vi "Stats to % Passing.vi"(11 "Stats by Ranking":T2) -> (3 "% Passing":T1)   [LabVIEW 2023, in "VIA Results Handling.lvlib"]
doc: "Converts stats by ranking into a % Passing by ranking."
uses:
  VIA Results Handling.lvlib
  Stats by Ranking.ctl
  Stats Cluster.ctl
  Ranking Percent Passing Cluster.ctl
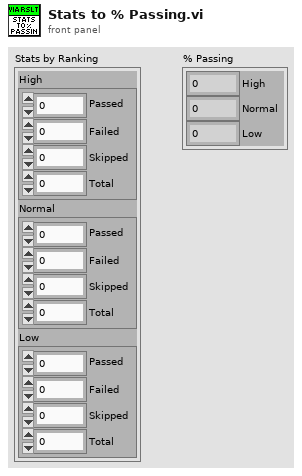
[diagram p1: front panel]
types:
  T1 = typedef "VIA Results Handling.lvlib/Ranking Percent Passing Cluster.ctl" = cluster{"High":dbl, "Normal":dbl, "Low":dbl}
  T2 = typedef "VIA Results Handling.lvlib/Stats by Ranking.ctl" = cluster{"High":T3, "Normal":T3, "Low":T3}
  T3 = typedef "VIA Results Handling.lvlib/Stats Cluster.ctl" = cluster{"Passed":i32, "Failed":i32, "Skipped":i32, "Total":i32}
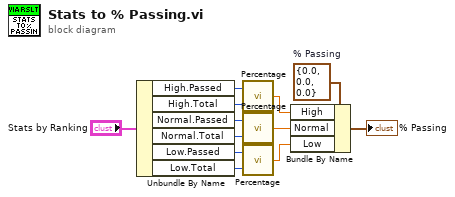
[diagram p0: block diagram]
diagram:
  w7 = T1 {"High"=0.0, "Normal"=0.0, "Low"=0.0}  # % Passing
  n1 = Unbundle By Name("Stats by Ranking") -> ("High.Passed"=w2:i32, "High.Total"=w1:i32, "Normal.Passed"=w3:i32, "Normal.Total"=w4:i32, "Low.Passed"=w5:i32, "Low.Total"=w6:i32)
  n2 = call "Percentage.vi"("A"=w1, "B"=w2) -> ("B/A (%)"=w9:dbl)
  n3 = call "Percentage.vi"("A"=w4, "B"=w3) -> ("B/A (%)"=w8:dbl)
  n4 = call "Percentage.vi"("A"=w6, "B"=w5) -> ("B/A (%)"=w10:dbl)
  n5 = Bundle By Name(cluster=w7, "High"=w9, "Normal"=w8, "Low"=w10) -> (→"% Passing":T1)
